vi "Get Input Script GainC(2).vi"(8 "error in (no error)":errorcluster, 10 "RxData Out":u16[](array[numeric]) format="%02d", 11 "Device Type":i32) -> (0 "error out":errorcluster, 2 "GAINC Input Error Code":string, 3 "GAINC Value":string)   [LabVIEW 2013]
uses:
  <vilib>/Utility/NIReport.llb/NI_report.lvclass
  InputScript states.ctl
  <vilib>/Utility/NIReport.llb/Excel/NI_Excel.lvclass
  <vilib>/addons/_office/NI_ReportGenerationToolkit.lvlib
  <vilib>/addons/_office/excel.llb/Excel Easy Table (str).vi
  <vilib>/addons/_office/excel.llb/Excel Get Data ([str]).vi
panel:
  out "output array":string[][](array[string])
  in  "State":T1
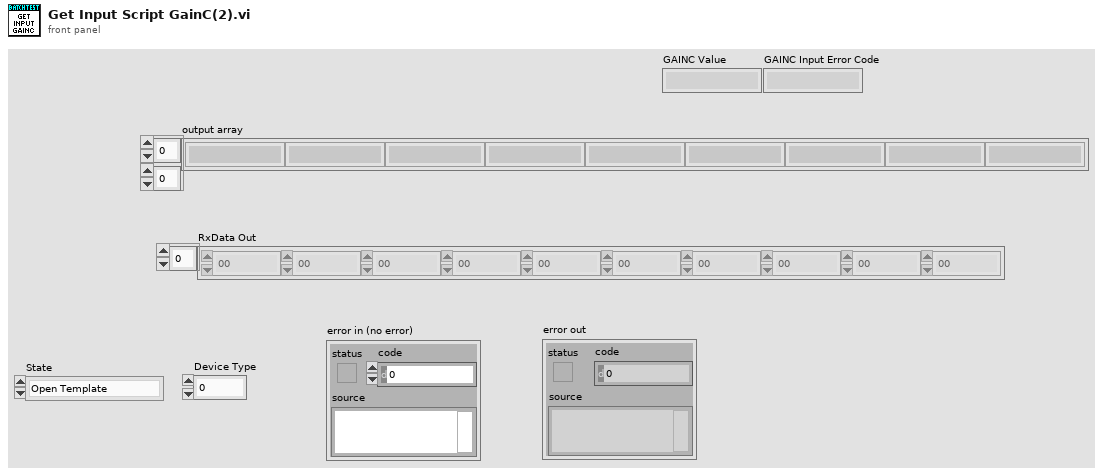
[diagram p1: front panel]
types:
  T1 = typedef "InputScript states.ctl" = enum16{"Open Template", "Setup parameters", "Read Input Script", "Close Template"}
  T2 = enum16{"Standard Report", "HTML", "Word", "Excel"}
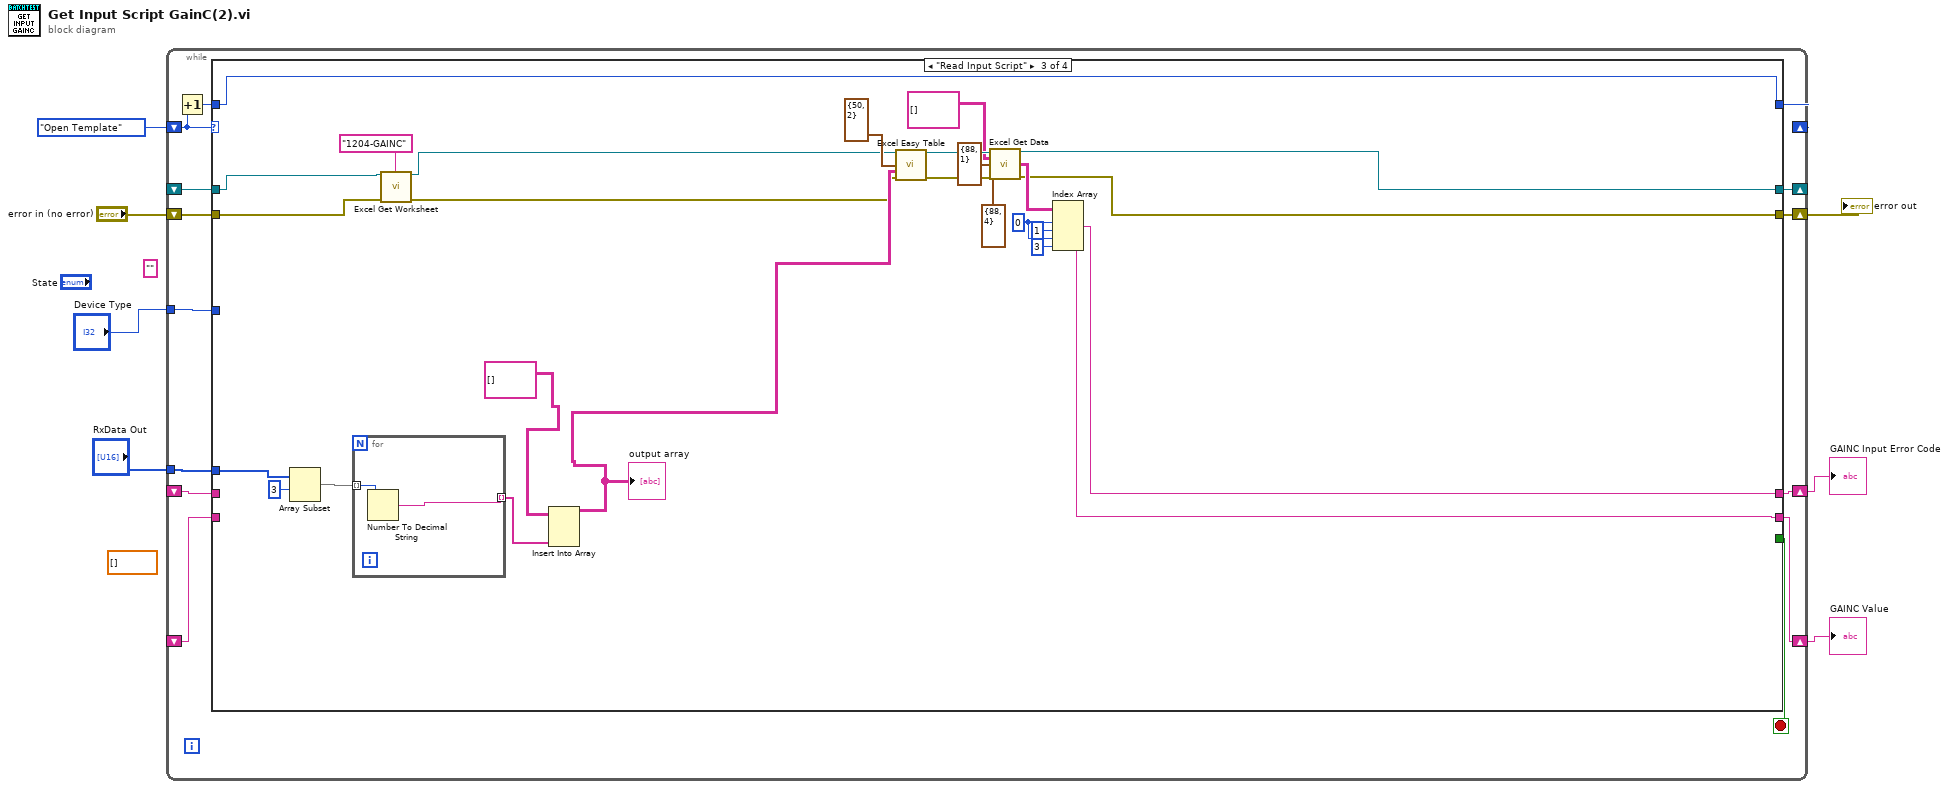
[diagram p0: block diagram]
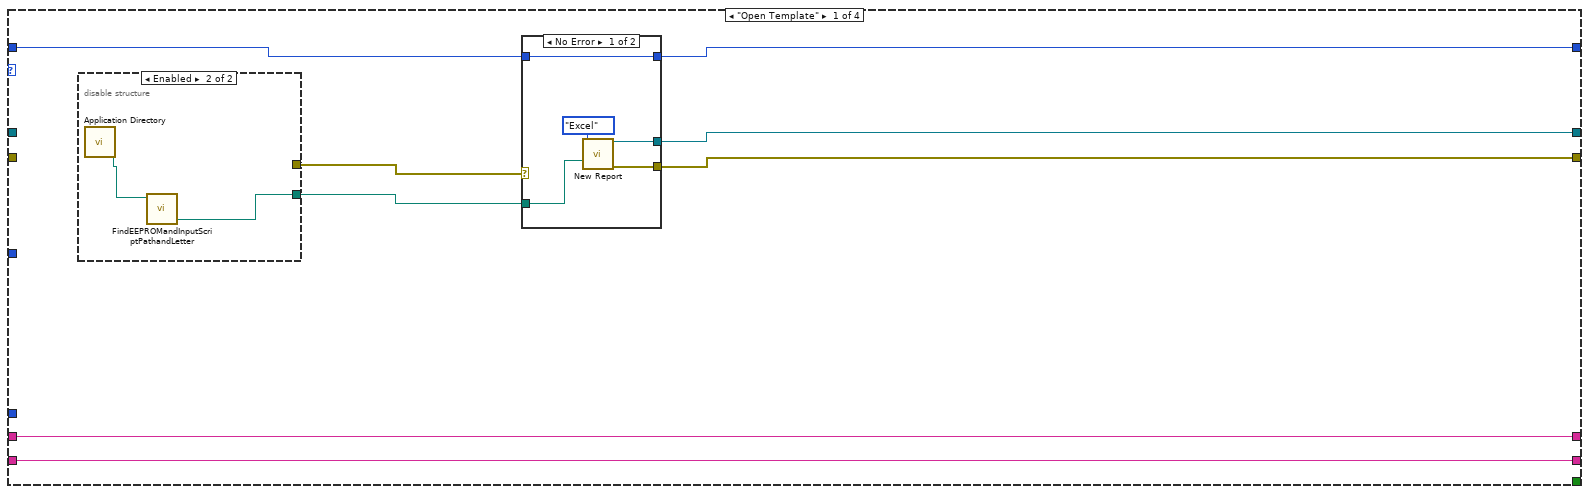
[diagram p2: hidden frame]
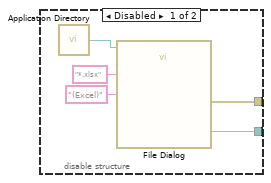
[diagram p3: hidden frame]
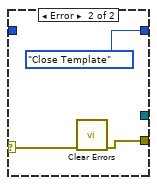
[diagram p4: hidden frame]
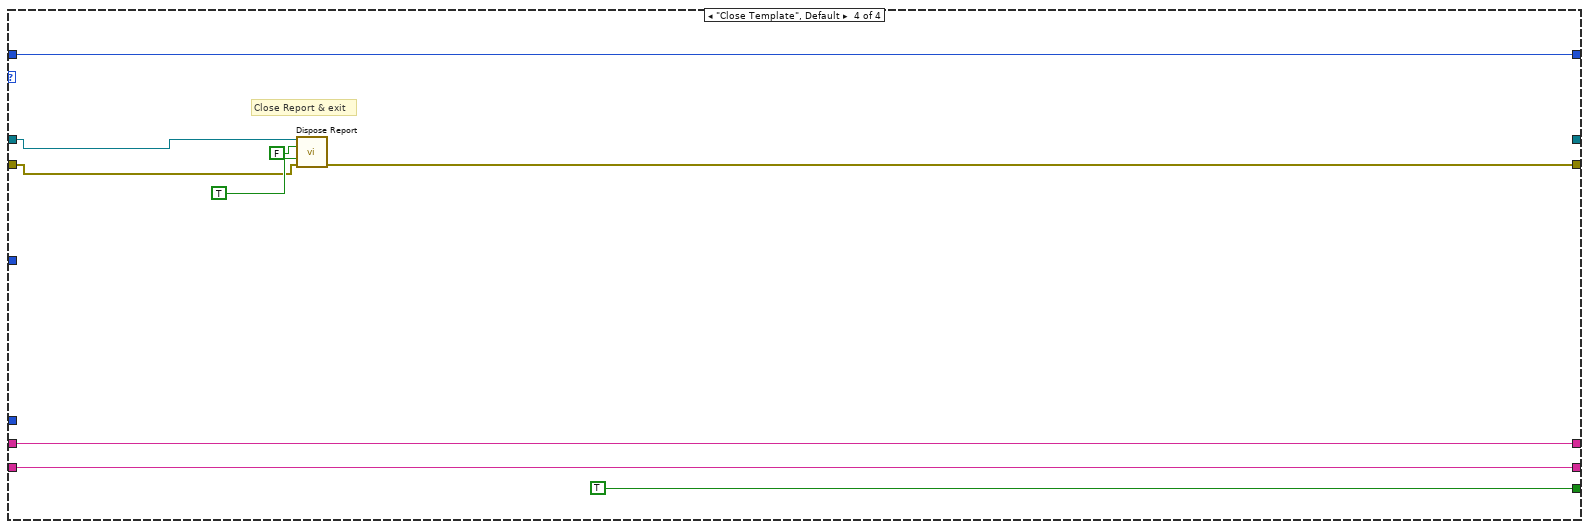
[diagram p6: hidden frame]
diagram:
  (unwired) dbl[] [] ("data")
  (unwired) "" ("Input Script Letter")
  n1 = while {
    shift-right: [w20] -> _
    shift-left: _ -> [w19]
    shift-right: [w18] -> w5
    shift-left: "error in (no error)" -> [w17]
    shift-right: [w14] -> _
    shift-left: InputScript_states."Open Template" -> [w16]
    tunnel: "Device Type" -> [w13]
    tunnel: "RxData Out" -> [w12]
    shift-right: [w9] -> w1
    shift-left: _ -> [w11]
    shift-right: [w8] -> w2
    shift-left: _ -> [w10]
    stop <- w21 stop-if-true
    n2 = Increment(x=w16) -> (x+1=w15:T1)
    n3 = case shown="\"Read Input Script\"" w16 {
      tunnel: [_ _ _ TRUE] -> w21
      tunnel: [w29 w49 w56 _] -> w20
      tunnel: w19 -> [_ w49 w61 w79]
      tunnel: [w28 w48 w55 w85] -> w18
      tunnel: w17 -> [_ w48 w60 w78]
      tunnel: w15 -> [w25 w47 w75 w83]
      tunnel: [w24 w47 w75 w83] -> w14
      tunnel: w13 -> [_ _ _ _]
      tunnel: w12 -> [_ _ w73 _]
      tunnel: [w22 w45 w50 w81] -> w8
      tunnel: [w23 w46 w51 w82] -> w9
      tunnel: w11 -> [w23 w46 _ w82]
      tunnel: w10 -> [w22 w45 _ w81]
      frame "Open Template" {
        n4 = disable-structure shown="Enabled" {
          disable-tunnel: [w31 w35] -> w27
          disable-tunnel: [w30 _] -> w26
          frame Disabled {
            n5 = call <vilib>:"Application Directory.vi"() -> ("Application Directory"=w32:path)
            n6 = call "File Dialog"("start path"=w32, "pattern (all files)"="*.xlsx", "pattern label"="(Excel)") -> ("selected path"=w31:path, "error out"=w30:errorcluster)  [unwired: 9 in, 2 out]
          }
          frame Enabled {
            n7 = call <vilib>:"Application Directory.vi"() -> ("Application Directory"=w36:path)
            n8 = call "FindEEPROMandInputScriptPathandLetter.vi"("path"=w36) -> ("Engineering Results File"=w35:path)  [unwired: 3 in, 3 out]
          }
        }
        n9 = case shown="No Error" w26 {
          selector: w26 -> [_ w44]
          tunnel: [w40 _] -> w29
          tunnel: [w39 w43] -> w28
          tunnel: w27 -> [w38 _]
          tunnel: w25 -> [w37 _]
          tunnel: [w37 InputScript_states."Close Template"] -> w24
          frame No Error {
            n10 = call <vilib>:"New Report.vi"("report type"=T2."Excel", "template (empty)"=w38) -> ("report out"=w40:refnum<class "NI_report.lvclass">, "error out"=w39:errorcluster)  [unwired: 12 in]
          }
          frame Error {
            n11 = call <vilib>:"Clear Errors.vi"("error in (no error)"=w44) -> ("error out"=w43:errorcluster)  [unwired: 5 in, 1 out]
          }
        }
      }
      frame "Setup parameters" {
      }
      frame "Read Input Script" {
        w54 = 0 ("index (row)")
        n12 = Array Subset(array=w73, index=3) -> (w70:u16[])  [unwired: 1 in]
        n13 = for {
          tunnel: w70 -> [w77] mode=indexing
          tunnel: [w76] -> w68 mode=indexing
          n14 = Number To Decimal String(number=w77) -> (decimal integer string=w76:string)  [unwired: 1 in]
        }
        n15 = call <vilib>:"Excel Get Worksheet.vi"("report in"=w61, "error in (no error)"=w60, "name (\"\")"="1204-GAINC" ("name (\"\")")) -> ("report out"=w59:refnum<class "NI_report.lvclass">, "error out"=w58:errorcluster)  [unwired: 11 in]
        n16 = Insert Into Array(array=string[][] [], new element=w68) -> (w67:string[][])  [unwired: 2 in]
        "output array" <- w67
        n17 = call-poly <vilib>:"Excel Easy Table.vi"("report in"=w59, "start (0, 0)"=cluster{"row":i32, "column":i32} {"row"=50, "column"=2}, "text data"=w67, "error in (no error)"=w58) -> ("report out"=w66:refnum<class "NI_report.lvclass">, "error out"=w65:errorcluster)  [unwired: 7 in, 3 out]
        n18 = call-poly <vilib>:"Excel Get Data.vi"("report in"=w66, "data type"=string[][] [], "start (-1, -1)"=cluster{"row":i32, "column":i32} {"row"=88, "column"=1}, "end (-1, -1)"=cluster{"row":i32, "column":i32} {"row"=88, "column"=4}, "error in (no error)"=w65) -> ("report out"=w56:refnum<class "NI_report.lvclass">, "data"=w57:string[][], "error out"=w55:errorcluster)  [unwired: 8 in]
        n19 = Index Array(array=w57, index (row) #1=w54, index (col) #1=1 ("disabled index (col)"), index (row) #2=w54, index (col) #2=3 ("disabled index (col)")) -> (element #1=w51:string, element #2=w50:string)
      }
      frame "Close Template", Default {
        # "Close Report & exit"
        n20 = call-dynamic "Dispose Report.vi"("report in"=w79, "wait until printing completed? (T)"=FALSE, "save changes? (F)"=TRUE, "error in (no error)"=w78) -> ("error out"=w85:errorcluster)  [unwired: 11 in]
      }
    }
  }
  "error out" <- w5
  "GAINC Input Error Code" <- w1
  "GAINC Value" <- w2
